vi "UHR-Fleezers Control (host) - 10.8.vi"() -> ()   [LabVIEW 2013] (continued)
  n124 = xnode "Read/Write Control"("FPGA VI Reference In"=w12, "error in"=w15, "Phase count adjustment"=w173, "Phase count adjustment (GI)"=w172, "Phase count adjustment (MCL)"=w171, "Phase Count Adjustment (APD Acq)"="Phase Adj. (APD Acq)", "Phase count adjustment (APD 1 Gate)"="Phase Adj. (APD 1 Gate)", "Phase count adjustment (APD 2 Gate)"="Phase Adj. (APD 2 Gate)", "Phase count adjustment (Green FB)"=w112, "Phase count adjustment (GI) 2"=w82) -> ("FPGA VI Reference Out"=w11:T19, "error out"=w10:errorcluster)
  n125 = call "Initialize RF boards - interlace 3.vi"("error in"=w10, "FPGA VI Reference In"=w11) -> ("FPGA VI Reference Out"=w149:T19)  [unwired: 1 out]
  n126 = call "set RF board frequency - interlace.vi"("Board 2 Frequency Limits"=w115, "Board 1 Frequency Limits"=w117, "FPGA VI Reference In"=w149, "Board 2 Frequency 3 (MHz)"="BD 2 Frequency 3 (MHz)", "Board 1 Frequency 3 (MHz)"="BD 1 Frequency 3 (MHz)", "Board 2 Frequency 2 (MHz)"="BD 2 Frequency 2 (MHz)", "Board 2 Frequency 1 (MHz)"="BD 2 Frequency 1 (MHz)", "Board 1 Frequency 2 (MHz)"="BD 1 Frequency 2 (MHz)", "Board 1 Frequency 1  (MHz)"="BD 1 Frequency 1 (MHz)") -> ("error out"=w243:errorcluster, "FPGA VI Reference Out"=w244:T19)  [unwired: 1 in]
  n127 = call "set RF board amplitude - interlace.vi"("Board 2 Amplitude Limits"=w114, "Board 1 Amplitude Limits"=w116, "error in"=w243, "FPGA VI Reference In"=w244, "Board 2 Amplitude 3 (%)"="BD 2 Amplitude 3 (%)", "Board 1 Amplitude 3 (%)"="BD 1 Amplitude 3 (%)", "Board 2 Amplitude 2 (%)"="BD 2 Amplitude 2 (%)", "Board 2 Amplitude 1 (%)"="BD 2 Amplitude 1 (%)", "Board 1 Amplitude 2 (%)"="BD 1 Amplitude 2 (%)", "Board 1 Amplitude 1 (%)"="BD 1 Amplitude 1 (%)") -> ("error out"=w8:errorcluster, "FPGA VI Reference Out"=w9:T19)
  n128 = flat-sequence {
    tunnel: w9 -> [w297]
    tunnel: w8 -> [w296]
    tunnel: [w295] -> w236
    tunnel: [w294] -> w235
    tunnel: [w301] -> w234
    tunnel: w236 -> [w301]
    tunnel: [w300] -> w233
    tunnel: w235 -> [w300]
    tunnel: w234 -> [w310]
    tunnel: w233 -> [w309]
    tunnel: [w308] -> w38
    tunnel: [w307] -> w37
    tunnel: w38 -> [w337]
    tunnel: w37 -> [w332]
    tunnel: [w337] -> w2
    tunnel: [w312] -> w1
    tunnel: [w338] -> w39
    tunnel: [w343] -> w16
    tunnel: w2 -> [w343]
    tunnel: w1 -> [w340]
    frame #0 {
      n129 = local read "Trap 1 (ON/OFF)"() -> (w289:bool)
      n130 = xnode "Read/Write Control"("FPGA VI Reference In"=w297, "error in"=w296, "Direct RF Box  Communication"=FALSE) -> ("FPGA VI Reference Out"=w295:T19, "error out"=w294:errorcluster)
      n131 = local write "Saving..."(FALSE ("Saving Data")) -> ()
      n132 = local write "Stop All"(FALSE ("Stop All")) -> ()
      n133 = local write "Index"(1.0 ("Index")) -> ()
      n134 = property on="Trap 1 ON" class="Bool (strict)"("Value"=w289) -> ()  [unwired: 2 in, 2 out]
      "Manipulating Trap" <- FALSE ("Manipulating Trap")
    }
    frame #1 {
      n135 = local read "Trap 2 (ON/OFF)"() -> (w299:bool)
      n136 = Wait (ms)(milliseconds to wait=u32 50) -> ()  [unwired: 1 out]
      n137 = property on="Trap 2 ON" class="Bool (strict)"("Val(Sgnl)"=w299) -> ()  [unwired: 2 in, 2 out]
    }
    frame #2 {
      n138 = local read "Scan Range (nm)"() -> (w303:dbl)
      n139 = xnode "Read/Write Control"("FPGA VI Reference In"=w310, "error in"=w309, "FPGA Controls  RF Box"=TRUE ("Direct RF Box  Communication")) -> ("FPGA VI Reference Out"=w308:T19, "error out"=w307:errorcluster)
      n140 = call "Update messages.vi"("Message to add"="UHR-Fleezers ready.", "Old message string"="") -> ("New message string"=w306:string)
      n141 = local write "Messages"(w306) -> ()
      n142 = property on="Scan Range (nm)" class="DigNum (strict)"("Val(Sgnl)"=w303) -> ()  [unwired: 2 in, 2 out]
    }
    frame #3 {
      w318 = T20."ASCII" ("Command")
      # "disable hysteresis\ncompensation for\nfaster performance"
      # "increase jerk\nfor faster \nresponse"
      # "disable backlash\ncompensation for\nfaster response \ntimes. necessary\nfor mouse control\nof stage"
      n143 = call "CONEX_FUNCTIONAL_GLOBAL.vi"("error in"=w332, "Command"=T20."INIT") -> ("error out"=w314:errorcluster)  [unwired: 7 in, 2 out]
      n144 = call "CONEX_FUNCTIONAL_GLOBAL.vi"("error in"=w314, "Position"=dbl[] [10.0, 12.0, 2.0], "Command"=T20."SET ULIM") -> ("error out"=w333:errorcluster)  [unwired: 6 in, 2 out]
      n145 = call "CONEX_FUNCTIONAL_GLOBAL.vi"("error in"=w333, "Position"=dbl[] [0.0, 0.0, 4.0], "Command"=T20."SET LLIM") -> ("error out"=w327:errorcluster)  [unwired: 6 in, 2 out]
      n146 = Concatenate Strings("1BA0", "\r\n") -> (w324:string)
      n147 = call "CONEX_FUNCTIONAL_GLOBAL.vi"("error in"=w327, "ASCII command"=w324, "Command"=w318) -> ("error out"=w323:errorcluster)  [unwired: 6 in, 2 out]
      n148 = Concatenate Strings("1JR0.001", "\r\n") -> (w320:string)
      n149 = call "CONEX_FUNCTIONAL_GLOBAL.vi"("error in"=w323, "ASCII command"=w320, "Command"=w318) -> ("error out"=w319:errorcluster)  [unwired: 6 in, 2 out]
      n150 = Concatenate Strings("1BH0", "\r\n") -> (w315:string)
      n151 = call "CONEX_FUNCTIONAL_GLOBAL.vi"("error in"=w319, "ASCII command"=w315, "Command"=w318) -> ("error out"=w313:errorcluster)  [unwired: 6 in, 2 out]
      n152 = call "CONEX_FUNCTIONAL_GLOBAL.vi"("error in"=w313, "Command"=T20."GET POS") -> ("error out"=w312:errorcluster, "Current Position"=w328:dbl[])  [unwired: 7 in, 1 out]
      n153 = local write "Current Position"(w328) -> ()
    }
    frame #4 {
      n154 = call "hamilton_controller.vi"("error in"=w340, "action"=T21."CONNECT") -> ("error out"=w339:errorcluster)  [unwired: 9 in]
      n155 = call "hamilton_controller.vi"("error in"=w339, "action"=T21."INITIALIZE VALVES") -> ("error out"=w338:errorcluster)  [unwired: 9 in]
    }
  }
  n156 = Subtract(x="BD 1 Frequency 1 (MHz)", y="BD 1 Frequency 2 (MHz)") -> (x-y=w159:dbl)
  n157 = Subtract(x="BD 2 Frequency 1 (MHz)", y="BD 2 Frequency 2 (MHz)") -> (x-y=w158:dbl)
  n158 = Square(x=w158) -> (x^2=w156:dbl)
  n159 = Square(x=w159) -> (x^2=w157:dbl)
  n160 = Add(x=w157, y=w156) -> (x+y=w155:dbl)
  n161 = Square Root(x=w155) -> (sqrt(x)=w154:dbl)
  n162 = local write "Trap Delta (MHz)"(w154) -> ()
  n163 = call "IMAQ Create"("Image Name"="APD 1 Image", "Image Type"=w63) -> ("New Image"=w62:T2)  [unwired: 3 in, 1 out]
  n164 = call "IMAQ Create"("Image Name"="APD 2 Image", "Image Type"=w63) -> ("New Image"=w61:T2)  [unwired: 3 in, 1 out]
  n165 = call "IMAQ Create"("Image Name"="Det. X Image", "Image Type"=w63) -> ("New Image"=w60:T2)  [unwired: 3 in, 1 out]
  n166 = call "IMAQ Create"("Image Name"="Det. Y Image", "Image Type"=w63) -> ("New Image"=w59:T2)  [unwired: 3 in, 1 out]
  n167 = Bundle("New Image"=w62, "New Image"=w61, "New Image"=w60, "New Image"=w59) -> (w58:T22)  [unwired: 1 in]
  n168 = disable-structure shown="Disabled" {
    disable-tunnel: w16 -> [w372 _]
    frame Disabled {
      w367 = T17 0 items=["Grayscale (U8)", "Grayscale (I16)", "Grayscale (SGL)", "Complex (CSG)", "RGB (U32)", "HSL (U32)", "RGB (U64)", "Grayscale (U16)"] ("Image Type")
      n169 = call <vilib>:"IMAQ Init.vi"("Interface Name"="img0") -> ("error out"=w369:errorcluster, "IMAQ Session Out"=w371:refnum<k11>)  [unwired: 9 in]
      n170 = call <vilib>:"IMAQ Grab Setup.vi"("error in (no error)"=w369, "IMAQ Session In"=w371) -> ("error out"=w365:errorcluster, "IMAQ Session Out"=w366:refnum<k11>)  [unwired: 8 in]
      n171 = call "IMAQ Create"("Image Name"="untitled", "Image Type"=w367) -> ("New Image"=w364:T2)  [unwired: 3 in, 1 out]
      n172 = call <vilib>:"Application Directory.vi"() -> ("Application Directory"=w351:path)
      n173 = Build Path(base path=w351, name or relative path="_trap_screen_positions") -> (appended path=w359:path)
      n174 = Open/Create/Replace File(file path (use dialog)=w359, operation (0:open)=T23."open or create", access (0:read/write)=enum16{"read/write", "read-only", "write-only"}."read/write") -> (refnum out=w361:refnum<file>)  [unwired: 3 in, 2 out]
      n175 = local read "Trap Sets"() -> (w353:u32)
      n176 = for "Load trap positions on video screen from file." {
        N: w353 -> [_]
        tunnel: [w379] -> w354
        tunnel: w361 -> [w378]
        tunnel: [w375] -> w350 mode=indexing
        w377 = 4
        n177 = for {
          N: w377 -> [_]
          tunnel: [w383] -> w379
          tunnel: w378 -> [w382]
          tunnel: w377 -> [w381]
          tunnel: [w380] -> w376 mode=indexing
          n178 = Read from Binary File(5:w381, 11:w382) -> (2:w380:i32, 3:w383:refnum<file>)  [unwired: 4 in, 2 out]
        }
        n179 = Array To Cluster(array=w376) -> (cluster=w375:T27)
      }
      n180 = node-c288() -> (w374:T24)  [unwired: 4 in]
      n181 = timed-loop "acquire video and stage position" {
        timing: w374 -> [_]
        timing-out: [_] -> w373
        tunnel: w366 -> [w402]
        tunnel: w365 -> [w401]
        tunnel: w364 -> [w400]
        tunnel: [w399] -> w346
        tunnel: [w396] -> w347
        tunnel: [w397] -> w345
        tunnel: w372 -> [_]
        shift-right: [w393] -> w363
        shift-left: w350 -> [w394]
        tunnel: w353 -> [w391]
        stop <- w398 stop-if-true
        n182 = node-c288() -> ()  [unwired: 1 in, 1 out]
        n183 = event shown="[2] \"Primary Video Display\": Mouse Down" {
          selector: _ -> [_ _ _ _]
          dyn-events: _ -> [_ _ _ _]
          timeout: 10 -> [_ _ _ _]
          tunnel: w402 -> [w413 w428 w437 w456]
          tunnel: w401 -> [w412 w430 w435 w458]
          tunnel: w400 -> [w411 w429 w436 w457]
          tunnel: [w410 w428 w437 w456] -> w399
          tunnel: [w403 w432 FALSE FALSE] -> w398
          tunnel: [w407 w430 w435 w458] -> w397
          tunnel: [w406 w429 w436 w457] -> w396
          tunnel: "radius" -> [_ _ w442 _]
          tunnel: w394 -> [w404 w431 w440 _]
          tunnel: [w404 w431 w441 cluster{i32, i32, i32, i32}[] []] -> w393
          tunnel: w391 -> [_ _ w433 _]
          event Timeout {
            n184 = event-data() -> ()  [unwired: 1 in, 2 out]
            n185 = call <vilib>:"IMAQ Grab Acquire.vi"("error in (no error)"=w412, "Image In"=w411, "IMAQ Session In"=w413) -> ("error out"=w408:errorcluster, "Image Out"=w409:T2, "IMAQ Session Out"=w410:refnum<k11>)  [unwired: 5 in, 1 out]
            n186 = case shown="True" "trap\nmarkers?" {
              tunnel: w404 -> [_ w421]
              tunnel: w409 -> [w415 w420]
              tunnel: w408 -> [w414 w419]
              tunnel: [w414 w418] -> w407
              tunnel: [w415 w416] -> w406
              frame False {
              }
              frame True {
                n187 = for {
                  tunnel: w421 -> [w427] mode=indexing
                  shift-right: [w425] -> w416
                  shift-left: w420 -> [w426]
                  tunnel: w419 -> [w424]
                  tunnel: [w423] -> w418
                  tunnel: u32 16711680 ("Color") -> [w422]
                  n188 = call "IMAQ Overlay Oval"("Color"=w422, "error in (no error)"=w424, "Bounding Rectangle"=w427, "Image"=w426) -> ("error out"=w423:errorcluster, "Image Out"=w425:T2)  [unwired: 6 in]
                }
              }
            }
            "Primary Video Display" <- w406
            n189 = Unbundle By Name(w408) -> ("status"=w403:bool)
          }
          event "Stop All": Value Change {
            n190 = event-data() -> ()  [unwired: 1 in, 5 out]
            n191 = local read "Stop All"() -> (w432:bool)
          }
          event "Primary Video Display": Mouse Down {
            n192 = event-data() -> ()  [unwired: 1 in, 7 out]
            n193 = Array Size(array=w440) -> (size(s)=w439:i32)
            n194 = Less?(x=w439, y=w433) -> (x < y?=w438:bool)
            n195 = case shown="True" w438 {
              tunnel: w442 -> [_ w452]
              tunnel: w440 -> [w443 w446]
              tunnel: [w443 w445] -> w441
              frame False {
              }
              frame True {
                n196 = property on="Primary Video Display" class="ImageControl"() -> ("Last Mouse Position"=w444:cluster{"X":i32, "Y":i32})  [unwired: 2 in, 2 out]
                n197 = Unbundle By Name(w444) -> ("X"=w454:i32, "Y"=w453:i32)
                n198 = Add(x=w453, y=w452) -> (x+y=w450:i32)
                n199 = Subtract(x=w453, y=w452) -> (x-y=w448:i32)
                n200 = Add(x=w454, y=w452) -> (x+y=w449:i32)
                n201 = Subtract(x=w454, y=w452) -> (x-y=w451:i32)
                n202 = Bundle(w451, w450, w449, w448) -> (w447:cluster{i32, i32, i32, i32})  [unwired: 1 in]
                n203 = Build Array (concatenate)(w446, w447) -> (w445:T28)
              }
            }
          }
          event "clear markers": Value Change {
            n204 = event-data() -> ()  [unwired: 1 in, 5 out]
          }
        }
        n205 = node-c288() -> ()  [unwired: 1 in, 1 out]
      }
      n206 = node-c288(w373) -> ()  [unwired: 1 out]
      n207 = Set File Position(offset (in bytes) (0)=i64 0, refnum=w354, from (0:start)=enum16{"start", "end", "current"}."start") -> (refnum out=w355:refnum<file>)  [unwired: 1 in, 1 out]
      n208 = for "Write trap positions to file so they can be remembered\nwhen program is removed from memory" {
        tunnel: w363 -> [w387] mode=indexing
        tunnel: [w385] -> w362
        tunnel: w355 -> [w384]
        n209 = Cluster To Array(cluster=w387) -> (array=w386:i32[])
        n210 = for {
          tunnel: w386 -> [w390] mode=indexing
          tunnel: [w389] -> w385
          tunnel: w384 -> [w388]
          n211 = Write to Binary File(file (use dialog)=w388, data=w390) -> (refnum out=w389:refnum<file>)  [unwired: 4 in, 2 out]
        }
      }
      n212 = Close File(refnum=w362) -> ()  [unwired: 1 in, 2 out]
      n213 = call "IMAQ Dispose"("Image"=w347, "error in (no error)"=w345) -> ("error out"=w344:errorcluster)  [unwired: 4 in]
      n214 = call <vilib>:"IMAQ Stop.vi"("error in (no error)"=w344, "IMAQ Session In"=w346) -> ("error out"=w348:errorcluster, "IMAQ Session Out"=w349:refnum<k11>)  [unwired: 8 in]
      n215 = call <vilib>:"IMAQ Close.vi"("error in (no error)"=w348, "IMAQ Session In"=w349) -> ()  [unwired: 9 in, 1 out]
    }
    frame Enabled {
    }
  }
  n216 = call <vilib>:"Initialize Mouse.vi"() -> ("error out"=w18:errorcluster, "device ID"=w19:refnum<k1>)  [unwired: 10 in]
  n217 = node-c288() -> (w4:T24)  [unwired: 4 in]
  n218 = call-poly <vilib>:"Acquire Input Data.vi"("device ID"=w19, "error in (no error)"=w18) -> ("device ID"=w20:refnum<k1>, "error out"=w17:errorcluster)  [unwired: 14 in, 2 out]
  n219 = timed-loop {
    tunnel: w20 -> [w471]
    tunnel: [w470] -> w21
    tunnel: [w469] -> _
    tunnel: w17 -> [w468]
    tunnel: w16 -> [_]
    shift-right: ["Use mouse to move stage\n(press mouse wheel to quit)"] -> _
    shift-left: _ -> [w465]
    timing: w4 -> [_]
    timing-out: [_] -> w3
    i -> [w464]
    stop <- w467 stop-if-true
    n220 = node-c288() -> ()  [unwired: 1 in, 1 out]
    n221 = case shown="False" "Use mouse to move stage\n(press mouse wheel to quit)" {
      tunnel: w471 -> [w481 w499]
      tunnel: [w481 w522] -> w470
      tunnel: [w474 w503] -> w469
      tunnel: w468 -> [w475 w497]
      tunnel: w465 -> [_ w500]
      tunnel: w464 -> [_ w495]
      frame False {
        n222 = case shown="True" "reset motor comm. link" {
          tunnel: [w482 w485] -> w476
          tunnel: w475 -> [w482 w484]
          frame False {
          }
          frame True {
            n223 = call "CONEX_FUNCTIONAL_GLOBAL.vi"("error in"=w484, "Command"=T20."CLOSE") -> ("error out"=w487:errorcluster)  [unwired: 7 in, 2 out]
            n224 = flat-sequence {
              tunnel: w487 -> [w490]
              tunnel: [w490] -> w486
              frame #0 {
                n225 = Wait (ms)(milliseconds to wait=u32 50) -> ()  [unwired: 1 out]
              }
            }
            n226 = local write "reset motor comm. link"(FALSE ("reset motor comm. link")) -> ()
            n227 = call "CONEX_FUNCTIONAL_GLOBAL.vi"("error in"=w486, "Command"=T20."INIT") -> ("error out"=w485:errorcluster)  [unwired: 7 in, 2 out]
          }
        }
        n228 = call "CONEX_FUNCTIONAL_GLOBAL.vi"("Axis"=enum16{"X", "Y", "Z", "XY", "XZ", "YZ", "XYZ"}."XYZ", "error in"=w476, "Command"=T20."GET POS") -> ("error out"=w474:errorcluster, "Current Position"=w478:dbl[])  [unwired: 6 in, 1 out]
        n229 = local write "Current Position"(w478) -> ()
      }
      frame True {
        # "put cursor somewhere\nwhere mouse clicks and \nmouse wheel moves won't\nbe heard by the window"
        n230 = Not(x=w500) -> (.not. x?=w501:bool)
        n231 = Quotient & Remainder(x=w495, y=10) -> (x-y*floor(x/y)=w493:i32)  [unwired: 1 out]
        n232 = case shown="True" w501 {
          tunnel: w499 -> [w526 w530]
          tunnel: [w526 w529] -> w498
          tunnel: w497 -> [w525 w528]
          tunnel: [w525 w527] -> w496
          frame False {
          }
          frame True {
            n233 = call-poly <vilib>:"Acquire Input Data.vi"("device ID"=w530, "error in (no error)"=w528) -> ("device ID"=w529:refnum<k1>, "error out"=w527:errorcluster)  [unwired: 14 in, 2 out]
          }
        }
        n234 = Equal To 0?(x=w493) -> (x = 0?=w492:bool)
        n235 = case shown="True" w492 {
          frame False {
          }
          frame True {
            # "SetCursorPos"
            n236 = dll-call lib="User32.dll" fn="SetCursorPos"(900, 600) -> ()  [unwired: 5 in, 3 out]
          }
        }
        n237 = call-poly <vilib>:"Acquire Input Data.vi"("device ID"=w498, "key mode"=enum16{"RELATIVE", "ABSOLUTE"}."RELATIVE", "error in (no error)"=w496) -> ("device ID"=w522:refnum<k1>, "axis info"=w520:T29, "error out"=w502:errorcluster)  [unwired: 13 in, 1 out]
        n238 = Cluster To Array(cluster=w520) -> (array=w518:i32[])
        n239 = Compound Arithmetic op=MULTIPLY(invert 10000.0 ("value"), "mouse sensitivity", w518) -> (w516:dbl[])
        n240 = call "subVI_explode3array.vi"("Array"=w516) -> ("x"=w507:dbl, "y"=w506:dbl, "z"=w515:dbl)  [unwired: 12 in]
        n241 = case shown="False" "invert y?" {
          tunnel: w506 -> [w531 w533]
          tunnel: [w531 w532] -> w505
          frame False {
          }
          frame True {
            n242 = Negate(x=w533) -> (-x=w532:dbl)
          }
        }
        n243 = case shown="False" "invert x?" {
          tunnel: w507 -> [w534 w536]
          tunnel: [w534 w535] -> w504
          frame False {
          }
          frame True {
            n244 = Negate(x=w536) -> (-x=w535:dbl)
          }
        }
        n245 = Divide(x=w515, y=50.0) -> (x/y=w513:dbl)
        n246 = Build Array(w504, w505, w513) -> (w510:dbl[])
        n247 = call "CONEX_FUNCTIONAL_GLOBAL.vi"("Axis"=enum16{"X", "Y", "Z", "XY", "XZ", "YZ", "XYZ"}."XYZ", "error in"=w502, "Position"=w510, "Command"=T20."REL MOVE") -> ("error out"=w503:errorcluster)  [unwired: 5 in, 2 out]
      }
    }
    n248 = local read "Stop All"() -> (w467:bool)
    n249 = node-c288() -> ()  [unwired: 1 in, 1 out]
  }
  n250 = node-c288(2 ("Processor")) -> (w7:T24)  [unwired: 3 in]
  n251 = node-c288() -> (w68:T24)  [unwired: 4 in]
  n252 = node-c288(i64 1 ("Period"), 1 ("Processor")) -> (w163:T24)  [unwired: 2 out]
  n253 = disable-structure shown="Enabled" {
    disable-tunnel: [w538 _] -> w32
    disable-tunnel: w16 -> [w537 _]
    frame Enabled {
      n254 = node-c288() -> (w540:T24)  [unwired: 4 out]
      n255 = timed-loop "Rough control of MCL mirror stage (debugging)" {
        tunnel: w537 -> [w543]
        tunnel: [w542] -> w538
        timing: w540 -> [_]
        timing-out: [_] -> w539
        stop <- w542 stop-if-true
        n256 = node-c288() -> ()  [unwired: 2 out]
        n257 = case shown="1" "MCL Mode" {
          tunnel: w543 -> [_ w546 w593]
          frame 0, Default {
            # "manual positioning"
          }
          frame 1 {
            # "sinusoidal wave"
            n258 = node-c288() -> (w548:T24)  [unwired: 4 out]
            n259 = timed-loop "Oscillate MCL mirror" {
              timing: w548 -> [_]
              timing-out: [_] -> w547
              tunnel: w546 -> [w587]
              i -> [w586]
              stop <- w549 stop-if-true
              n260 = node-c288() -> (w585:i64)  [unwired: 1 out]
              n261 = Multiply(x="AO1", y=32767.0) -> (x*y=w581:dbl)
              n262 = Multiply(x="AO2", y=32767.0) -> (x*y=w576:dbl)
              n263 = Divide(x=w581, y=10.0) -> (x/y=w582:dbl)
              n264 = Divide(x=w576, y=10.0) -> (x/y=w577:dbl)
              n265 = To Word Integer(number=w582) -> (16bit integer=w574:i16)
              n266 = To Word Integer(number=w577) -> (16bit integer=w573:i16)
              n267 = Divide(x=w585, y=i64 1000) -> (x/y=w556:dbl)
              n268 = Multiply(x=w556, y=w586) -> (x*y=w567:dbl)
              n269 = Multiply(x="Osc. freq. (Hz) 2", y=6.283185307179586) -> (x*y=w568:dbl)
              n270 = Multiply(x=w568, y=w567) -> (x*y=w566:dbl)
              n271 = Sine(x=w566) -> (sin(x)=w565:dbl)
              n272 = Multiply(x=w565, y="Osc. amp. (V)") -> (x*y=w563:dbl)
              n273 = Add(x=w563, y="Osc. center (V)") -> (x+y=w561:dbl)
              n274 = Divide(x=w561, y=10.0) -> (x/y=w559:dbl)
              n275 = Multiply(x=w559, y=32767.0) -> (x*y=w554:dbl)
              n276 = Select(t=w554, s="Scan axis", f=w574) -> (s? t:f=w572:dbl)
              n277 = Select(t=w573, s="Scan axis", f=w554) -> (s? t:f=w571:dbl)
              n278 = local read "MCL Mode"() -> (w553:u16)
              n279 = Not Equal?(x=w553, y=u16 1) -> (x != y?=w550:bool)
              n280 = local read "Stop All"() -> (w551:bool)
              n281 = xnode "Read/Write Control"("FPGA VI Reference In"=w587, "AO1"=w572, "AO2"=w571) -> ()  [unwired: 1 in, 2 out]
              n282 = Compound Arithmetic op=OR(w551, w550) -> (w549:bool)
              n283 = node-c288() -> ()  [unwired: 2 out]
            }
            n284 = node-c288(w547) -> ()  [unwired: 1 out]
          }
          frame 2 {
            # "linear scan"
            n285 = case shown="True" "Start Scan" {
              tunnel: w593 -> [_ w605]
              frame False {
              }
              frame True {
                n286 = Subtract(x="End (V)", y="Begin (V)") -> (x-y=w601:dbl)
                n287 = Decrement(x="N Points") -> (x-1=w600:dbl)
                n288 = Divide(x=w601, y=w600) -> (x/y=w598:dbl)
                n289 = for {
                  N: "N Points" -> [_]
                  tunnel: "Begin (V)" -> [w618]
                  tunnel: w605 -> [w610]
                  tunnel: [w609] -> w604 mode=indexing
                  tunnel: w598 -> [w608]
                  tunnel: [w606] -> w597 mode=indexing
                  i -> [w617]
                  n290 = Multiply(x=w608, y=w617) -> (x*y=w616:dbl)
                  n291 = Add(x=w618, y=w616) -> (x+y=w613:dbl)
                  n292 = local read "Scan axis"() -> (w607:bool)
                  n293 = local read "AO1"() -> (w615:dbl)
                  n294 = local read "AO2"() -> (w614:dbl)
                  n295 = Select(t=w613, s=w607, f=w615) -> (s? t:f=w612:dbl)
                  n296 = Select(t=w614, s=w607, f=w613) -> (s? t:f=w611:dbl)
                  n297 = flat-sequence {
                    tunnel: w612 -> [w622]
                    tunnel: w611 -> [w621]
                    tunnel: w610 -> [w619]
                    tunnel: [w632] -> w609
                    tunnel: [w631] -> w606
                    frame #0 {
                      w625 = 10.0 ("y")
                      w620 = 32767.0 ("y")
                      n298 = Multiply(x=w622, y=w620) -> (x*y=w628:dbl)
                      n299 = Multiply(x=w621, y=w620) -> (x*y=w626:dbl)
                      n300 = Divide(x=w628, y=w625) -> (x/y=w629:dbl)
                      n301 = Divide(x=w626, y=w625) -> (x/y=w627:dbl)
                      n302 = To Word Integer(number=w629) -> (16bit integer=w623:i16)
                      n303 = To Word Integer(number=w627) -> (16bit integer=w624:i16)
                      n304 = xnode "Read/Write Control"("FPGA VI Reference In"=w619, "AO1"=w623, "AO2"=w624) -> ()  [unwired: 1 in, 2 out]
                    }
                    frame #1 {
                      n305 = Wait (ms)(milliseconds to wait="DAQ Delay (ms)") -> ()  [unwired: 1 out]
                    }
                    frame #2 {
                      n306 = local read "Slow mean"() -> (w632:dbl)
                      n307 = local read "Sigma"() -> (w631:dbl)
                    }
                  }
                }
                n308 = Bundle("Begin (V)"="Begin (V)", w598, w604) -> (→"MCL Scan":cluster{"Begin (V)":dbl, dbl, dbl[]})  [unwired: 1 out]
                n309 = Bundle("Begin (V)"="Begin (V)", w598, w597) -> (→"MCL Scan 2":cluster{"Begin (V)":dbl, dbl, dbl[]})  [unwired: 1 out]
              }
            }
          }
        }
        n310 = local read "Stop All"() -> (w542:bool)
        n311 = node-c288() -> ()  [unwired: 2 out]
      }
      n312 = node-c288(w539) -> ()  [unwired: 1 out]
    }
    frame Disabled {
    }
  }
  n313 = timed-loop "Control parameters (event loop)" {
    tunnel: w16 -> [w638]
    shift-right: [w637] -> _
    shift-left: errorcluster {"status"=FALSE, "code"=0, "source"=""} ("error out") -> [w636]
    tunnel: [w635] -> w34
    timing: w7 -> [_]
    timing-out: [_] -> w6
    stop <- w635 stop-if-true
    n314 = node-c288() -> ()  [unwired: 1 in, 1 out]
    n315 = event shown="[32] \"Raster Scanning...\": Value Change" {
      selector: _ -> [_ _ _ _ _ _ _ _ _ _ _ _ _ _ _ _ _ _ _ _ _ _ _ _ _ _ _ _ _ _ _ _ _ _ _ _ _ _ _ _ _ _ _ _ _ _ _ _ _ _ _ _ _ _ _ _ _]
      dyn-events: _ -> [_ _ _ _ _ _ _ _ _ _ _ _ _ _ _ _ _ _ _ _ _ _ _ _ _ _ _ _ _ _ _ _ _ _ _ _ _ _ _ _ _ _ _ _ _ _ _ _ _ _ _ _ _ _ _ _ _]
      timeout: _ -> [_ _ _ _ _ _ _ _ _ _ _ _ _ _ _ _ _ _ _ _ _ _ _ _ _ _ _ _ _ _ _ _ _ _ _ _ _ _ _ _ _ _ _ _ _ _ _ _ _ _ _ _ _ _ _ _ _]
      tunnel: w638 -> [w676 _ _ _ w713 _ w735 _ w799 _ _ _ w842 _ _ w885 w891 w896 w902 w938 w956 w963 _ w981 w992 w1003 w1014 w1025 w1036 w1054 w1060 w1154 _ w1163 w1201 _ _ w1300 w1304 w1315 w1319 w1323 _ w1331 _ _ _ _ w1465 _ w1482 w1485 w1494 w1497 w1501 _ w1518]
      tunnel: [w675 _ _ _ w703 _ w734 _ w762 _ w807 _ w821 _ _ w884 w887 w893 w899 w937 w954 w962 _ w975 w986 w997 w1008 w1019 w1030 w1052 w1059 w1152 _ w1161 w1199 _ _ w1298 w1302 w1305 w1317 w1321 _ w1329 _ _ _ _ w1463 _ _ _ _ _ _ _ _] -> w637
      tunnel: w636 -> [w674 _ _ _ w712 _ w733 _ w794 _ w807 _ w841 _ _ w883 w886 w892 w898 w936 w955 w961 _ w980 w991 w1002 w1013 w1024 w1035 w1053 w1058 w1153 _ w1162 w1200 _ _ w1299 w1303 w1314 w1318 w1322 _ w1330 _ _ _ _ w1464 _ w1481 w1484 w1493 w1496 w1500 _ w1517]
      tunnel: [_ _ _ _ _ _ _ _ _ _ w806 _ _ _ _ _ _ _ _ _ _ _ _ _ _ _ _ _ _ _ _ _ _ _ _ _ _ _ _ _ _ _ _ _ _ _ _ _ _ _ _ _ _ _ _ _ _] -> w635
      tunnel: [_ _ _ _ _ _ _ "Round T1 X" _ _ _ _ _ _ _ _ _ _ _ _ _ _ _ _ _ _ _ _ _ _ _ _ _ _ _ _ _ _ _ _ _ _ _ _ _ _ _ _ _ _ _ _ _ _ _ _ _] -> _
      tunnel: [_ _ _ "Adjust Scale\nto Mean" _ _ _ _ _ _ _ _ _ _ _ _ _ _ _ _ _ _ _ _ _ _ _ _ _ _ _ _ _ _ _ _ _ _ _ _ _ _ _ _ _ _ _ _ _ _ _ _ _ _ "Set SP to Reading" _ _] -> _
      tunnel: [_ _ _ _ _ _ _ _ _ "Round T2 X" _ "Delayed Interlace Start" _ _ _ _ _ _ _ _ _ _ _ _ _ _ _ _ _ _ _ _ _ _ _ _ _ _ _ _ _ _ _ _ _ _ _ _ _ _ _ _ _ _ _ _ _] -> _
      event "AI Count (ticks)", "Sets to FIFO (Traps)", "Save ave N", "FPGA Ave.", "# Samples/channel", "N sets to save": Value Change {
        # "So that if 'Save ave N' is updated, the AOD scanning code updates too."
        n316 = event-data() -> ()  [unwired: 6 out]
        n317 = local read "AI Count (ticks)"() -> (w656:u32)
        n318 = Boolean To (0,1)(Boolean="Sets to FIFO (Traps)") -> (0, 1=w666:cluster{"Set 1":i16, "Set 2":i16, "Set 3":i16})
        n319 = xnode "Read/Write Control"("FPGA VI Reference In"=w676, "error in"=w674, "ai count"=w656, "AI1 Sets to FIFO"="Sets to FIFO (Traps)", "N of AI1 Int Acq Sets"="N Acq Sets (Traps + Fl.)") -> ("error out"=w675:errorcluster)  [unwired: 1 out]
        n320 = Cluster To Array(cluster=w666) -> (array=w665:i16[])
        n321 = To Unsigned Long Integer(number=w665) -> (unsigned 32bit integer=w645:u32[])
        n322 = local read "Scan steps (AOD)"() -> (w667:u64)
        n323 = Multiply(x=w656, y="N Acq Sets (Traps + Fl.)") -> (x*y=w654:u32)
        n324 = Divide(x=40000000.0, y=w656) -> (x/y=w648:dbl)
        "AI rate (Hz)" <- w648
        "Ave. Rate (Hz)" <- w648
        n325 = Add Array Elements(numeric array=w645) -> (sum=w657:u32)
        "Trap Sets" <- w657
        n326 = Reciprocal(x=w648) -> (1/x=→"Ave. Period (s)":dbl)
        n327 = property on="Scan steps (AOD)" class="DigNum (strict)"("Val(Sgnl)"=w667) -> ()  [unwired: 2 in, 2 out]
        n328 = Divide(x=w648, y="N Acq Sets (Traps + Fl.)") -> (x/y=w671:dbl)
        "Data Rate (Hz)" <- w671
        n329 = Reciprocal(x=w671) -> (1/x=→"Data Period (s)":dbl)
        n330 = local read "Save ave N"() -> (w670:dbl)
        n331 = Divide(x=w671, y=w670) -> (x/y=w669:dbl)
        "Save Data Rate (Hz)" <- w669
        n332 = Reciprocal(x=w669) -> (1/x=→"Save Data Period (s)":dbl)
        n333 = Multiply(x=w654, y="# Samples/trap") -> (x*y=w652:u32)
        "Counts/DMA" <- w652
        n334 = property on="Trap Disp. Downsample" class="DigNum (strict)"("Maximum"="# Samples/trap") -> ()  [unwired: 2 in, 2 out]
        n335 = Multiply(x=w657, y="# Samples/trap") -> (x*y=w646:u32)
        "# Samples/channel" <- w646
        n336 = Multiply(x=w646, y=u32 8) -> (x*y=→"Trap AI Elements/DMA read":u32)
        n337 = local read "APD Int. Count"() -> (w653:u32)
        n338 = Multiply(x=w646, y=u32 3) -> (x*y=→"Trap Pos Elements/DMA read":u32)
        n339 = Divide(x=w652, y=w653) -> (x/y=w643:dbl)
        "APD Samples/FIFO Acq." <- w643
        n340 = Divide(x=w652, y=40000000.0) -> (x/y=w650:dbl)
        "DMA Update Period (s)" <- w650
        n341 = Multiply(x=2.0, y=w643) -> (x*y=→"APD Elements/DMA read":dbl)
        n342 = property on="APD Disp. Downsample" class="DigNum (strict)"("Maximum"=w643) -> ()  [unwired: 2 in, 2 out]
        n343 = local read "N sets to save"() -> (w663:u32)
        n344 = Multiply(x=w650, y=w663) -> (x*y=→"Total Time (s)":dbl)
        "FPGA Averaging" <- FALSE ("FPGA Averaging")
      }
      event "Rescale on Mean": Value Change {
        n345 = event-data() -> ()  [unwired: 7 out]
        n346 = And(x=FALSE, y="Rescale on Mean") -> (x .and. y?=w678:bool)
        n347 = local write "Rescale on Mean"(w678) -> ()
        n348 = local read "Bead Mean (nm)"() -> (w683:dbl)
        n349 = Add(x="Amplitude (nm)", y=w683) -> (x+y=w681:dbl)
        n350 = Subtract(x=w683, y="Amplitude (nm)") -> (x-y=w680:dbl)
        n351 = property on="Bead Separation" class="WFChart (strict)"("YScale.Minimum"=w680) -> ()  [unwired: 2 in, 2 out]
        n352 = property on="Bead Separation" class="WFChart (strict)"("YScale.Maximum"=w681) -> ()  [unwired: 2 in, 2 out]
      }
      event "Detector Type": Value Change {
        n353 = event-data() -> ()  [unwired: 7 out]
        n354 = local read "AI labels"() -> (w684:string[])
        n355 = property on="High Res. Display" class="Ring (strict)"("Strings []"=w684) -> ()  [unwired: 2 in, 2 out]
        n356 = Build Array (concatenate)(w684, "none") -> (w685:string[])
        n357 = property on="FFT 1 Choice 1" class="Ring (strict)"("Strings []"=w685) -> ()  [unwired: 2 in, 2 out]
        n358 = property on="FFT 1 Choice 2" class="Ring (strict)"("Strings []"=w685) -> ()  [unwired: 2 in, 2 out]
        n359 = property on="FFT 2 Choice 1" class="Ring (strict)"("Strings []"=w685) -> ()  [unwired: 2 in, 2 out]
        n360 = property on="FFT 2 Choice 2" class="Ring (strict)"("Strings []"=w685) -> ()  [unwired: 2 in, 2 out]
        n361 = Bundle("APD 1", "APD 2") -> (w688:cluster{string, string})  [unwired: 1 out]
        n362 = Cluster To Array(cluster=w688) -> (array=w686:string[])
        n363 = Build Array (concatenate)(w686, w685) -> (w690:string[])
        n364 = Array Size(array=w690) -> (size(s)=w691:i32)
        n365 = property on="Signals to Plot" class="LstBox (strict)"("Item Names"=w690) -> ()  [unwired: 2 in, 2 out]
        n366 = property on="Signals to Plot" class="LstBox (strict)"("Number of Rows"=w691) -> ()  [unwired: 2 in, 2 out]
        n367 = property on="All Signals" class="WFChart (strict)"("LegNumRows"=w691) -> ()  [unwired: 2 in, 2 out]
      }
      event "Adjust Scale\nto Mean": Value Change {
        n368 = event-data() -> ()  [unwired: 7 out]
        n369 = local read "APD 1 Rate (Hz)"() -> (w700:dbl)
        n370 = Multiply(x=1000.0, y="Above (kHz)") -> (x*y=w698:dbl)
        n371 = Multiply(x=1000.0, y="Below (kHz)") -> (x*y=w696:dbl)
        n372 = Add(x=w698, y=w700) -> (x+y=w693:dbl)
        n373 = Subtract(x=w700, y=w696) -> (x-y=w694:dbl)
        n374 = property on="APD Chart" class="WFChart (strict)"("YScale.Minimum"=w694) -> ()  [unwired: 2 in, 2 out]
        n375 = property on="APD Chart" class="WFChart (strict)"("YScale.Maximum"=w693) -> ()  [unwired: 2 in, 2 out]
      }
      event "Phase adj. (AI1)", "+ phase (AI1)", "- phase (AI1)": Value Change {
        n376 = event-data() -> ()  [unwired: 7 out]
        n377 = Negate(x="Phase adj. (AI1)") -> (-x=w710:i16)
        n378 = Select(t=w710, s="- phase (AI1)", f="Phase adj. (AI1)") -> (s? t:f=w709:i16)
        n379 = xnode "Read/Write Control"("FPGA VI Reference In"=w713, "error in"=w712, "Phase count adjustment"=w709) -> ("FPGA VI Reference Out"=w708:T19, "error out"=w707:errorcluster)
        n380 = Or(x="- phase (AI1)", y="+ phase (AI1)") -> (x .or. y?=w704:bool)
        n381 = xnode "Read/Write Control"("FPGA VI Reference In"=w708, "error in"=w707, "+ phase"=w704) -> ("error out"=w703:errorcluster)  [unwired: 1 out]
      }
      event "Signals to Plot": Double Click {
        w716 = u32 9868950 ("Color Box")
        n382 = event-data() -> ("Row"=w718:i32)  [unwired: 9 out]
        n383 = property on="All Signals" class="WFChart (strict)"("Active Plot"=w718) -> (error out=w729:errorcluster)  [unwired: 2 in, 1 out]
        n384 = property on="All Signals" class="WFChart (strict)" props=["Plot", "Visible?", "Plot", "Plot Color"](error in=w729) -> (error out=w728:errorcluster, "Plot.Visible?"=w727:bool)  [unwired: 1 in, 2 out]
        n385 = Select(t=FALSE ("Plot.Visible"), s=w727, f=TRUE ("Plot.Visible")) -> (s? t:f=w722:bool)
        n386 = property on="All Signals" class="WFChart (strict)"(error in=w728, "Plot.Visible?"=w722) -> (error out=w724:errorcluster)  [unwired: 1 in, 1 out]
        n387 = property on="All Signals" class="WFChart (strict)"(error in=w724) -> (error out=w719:errorcluster, "Plot.Plot Color"=w723:u32)  [unwired: 1 in, 1 out]
        n388 = property on="Signals to Plot" class="LstBox (strict)"(error in=w719, "Active Row"=w718) -> (error out=w717:errorcluster)  [unwired: 1 in, 1 out]
        n389 = Select(t=w723, s=w722, f=u32 0) -> (s? t:f=w720:u32)
        n390 = property on="Signals to Plot" class="LstBox (strict)"(error in=w717, "CellFontColor"=w720, "SelColor"=w716, "CellBG"=w716, "CellFontSize"=u32 20 ("Active Row:Cell Font:Size"), "CellFontBold"=TRUE ("Active Row:Cell Font:Bold")) -> ()  [unwired: 1 in, 2 out]
      }
      event "BD 1 Frequency 1 (MHz)", "BD 1 Frequency 2 (MHz)", "BD 1 Frequency 3 (MHz)", "BD 2 Frequency 1 (MHz)", "BD 2 Frequency 2 (MHz)", "BD 2 Frequency 3 (MHz)", "Trap Delta (MHz)": Value Change {
        # "anytime one of the frequencies is changed, write it to the RF board UNLESS Set 2 is being oscillated. The oscillation\nscript writes the frequencies to the RF board."
        n391 = event-data() -> ("CtlRef"=w732:refnum<vi>)  [unwired: 6 out]
        n392 = control-ref of="Trap Delta (MHz)"() -> (w731:refnum<vi>)
        n393 = Equal?(x=w731, y=w732) -> (x = y?=w730:bool)
        n394 = case shown="False" "Oscillate Set 2" {
          tunnel: w735 -> [w755 _]
          tunnel: [w754 w758] -> w734
          tunnel: w733 -> [w753 w758]
          tunnel: w730 -> [w739 _]
          frame False {
            n395 = local read "BD 1 Frequency 1 (MHz)"() -> (w737:dbl)
            n396 = local read "BD 1 Frequency 2 (MHz)"() -> (w741:dbl)
            n397 = Add(x=w737, y="Trap Delta (MHz)") -> (x+y=w740:dbl)
            n398 = Select(t=w740, s=w739, f=w741) -> (s? t:f=w738:dbl)
            n399 = local read "Y RF Frequency Limits (MHz)"() -> (w743:T16)
            n400 = local read "X RF Frequency Limits (MHz)"() -> (w744:T16)
            n401 = local read "BD 1 Frequency 3 (MHz)"() -> (w756:dbl)
            n402 = local write "BD 1 Frequency 2 (MHz)"(w738) -> ()
            n403 = local read "BD 2 Frequency 1 (MHz)"() -> (w747:dbl)
            n404 = local read "BD 2 Frequency 2 (MHz)"() -> (w746:dbl)
            n405 = local read "BD 2 Frequency 3 (MHz)"() -> (w757:dbl)
            n406 = call "set RF board frequency - interlace.vi"("Board 2 Frequency Limits"=w743, "Board 1 Frequency Limits"=w744, "error in"=w753, "FPGA VI Reference In"=w755, "Board 2 Frequency 3 (MHz)"=w757, "Board 1 Frequency 3 (MHz)"=w756, "Board 2 Frequency 2 (MHz)"=w746, "Board 2 Frequency 1 (MHz)"=w747, "Board 1 Frequency 2 (MHz)"=w738, "Board 1 Frequency 1  (MHz)"=w737) -> ("error out"=w754:errorcluster)  [unwired: 1 out]
            n407 = Subtract(x=w747, y=w746) -> (x-y=w751:dbl)
            n408 = Subtract(x=w738, y=w737) -> (x-y=w752:dbl)
            n409 = Square(x=w751) -> (x^2=w749:dbl)
            n410 = Square(x=w752) -> (x^2=w750:dbl)
            n411 = Add(x=w750, y=w749) -> (x+y=w748:dbl)
            n412 = Square Root(x=w748) -> (sqrt(x)=w745:dbl)
            n413 = local write "Trap Delta (MHz)"(w745) -> ()
            n414 = property on="Initial delta (MHz)" class="DigNum (strict)"("Val(Sgnl)"=w745) -> ()  [unwired: 2 in, 2 out]
          }
          frame True {
          }
        }
      }
      event "Round T1 X": Value Change {
        n415 = event-data() -> ()  [unwired: 7 out]
        n416 = local read "BD 1 Frequency 1 (MHz)"() -> (w761:dbl)
        n417 = Round To Nearest(number=w761) -> (nearest integer value=w760:dbl)
        n418 = property on="BD 1 Frequency 1 (MHz)" class="DigNum (strict)"("Val(Sgnl)"=w760) -> ()  [unwired: 2 in, 2 out]
      }
      event "Restart RF": Value Change {
        n419 = event-data() -> ()  [unwired: 7 out]
        n420 = xnode "Read/Write Control"("FPGA VI Reference In"=w799, "error in"=w794, "FPGA Controls  RF Box"=FALSE) -> ("FPGA VI Reference Out"=w798:T19, "error out"=w793:errorcluster)
        n421 = local read "Y RF Amplitude Limits (%)"() -> (w774:T16)
        n422 = local read "X RF Amplitude Limits (%)"() -> (w775:T16)
        n423 = local read "X RF Frequency Limits (MHz)"() -> (w777:T16)
        n424 = local read "Y RF Frequency Limits (MHz)"() -> (w776:T16)
        n425 = xnode "Read/Write Control"("FPGA VI Reference In"=w798, "error in"=w793, "Direct RF Box  Communication"=TRUE) -> ("FPGA VI Reference Out"=w797:T19, "error out"=w792:errorcluster)
        n426 = local read "BD 2 Frequency 3 (MHz)"() -> (w784:dbl)
        n427 = local read "BD 2 Frequency 2 (MHz)"() -> (w785:dbl)
        n428 = local read "BD 1 Frequency 3 (MHz)"() -> (w788:dbl)
        n429 = local read "BD 1 Frequency 1 (MHz)"() -> (w789:dbl)
        n430 = local read "BD 2 Frequency 1 (MHz)"() -> (w786:dbl)
        n431 = local read "BD 1 Frequency 2 (MHz)"() -> (w787:dbl)
        n432 = call "Initialize RF boards - interlace 3.vi"("error in"=w792, "FPGA VI Reference In"=w797) -> ("error out"=w791:errorcluster, "FPGA VI Reference Out"=w796:T19)
        n433 = local read "BD 2 Amplitude 2 (%)"() -> (w779:dbl)
        n434 = local read "BD 2 Amplitude 1 (%)"() -> (w780:dbl)
        n435 = local read "BD 2 Amplitude 3 (%)"() -> (w778:dbl)
        n436 = local read "BD 1 Amplitude 3 (%)"() -> (w783:dbl)
        n437 = local read "BD 1 Amplitude 1 (%)"() -> (w782:dbl)
        n438 = local read "BD 1 Amplitude 2 (%)"() -> (w781:dbl)
        n439 = call "set RF board frequency - interlace.vi"("Board 2 Frequency Limits"=w776, "Board 1 Frequency Limits"=w777, "error in"=w791, "FPGA VI Reference In"=w796, "Board 2 Frequency 3 (MHz)"=w784, "Board 1 Frequency 3 (MHz)"=w788, "Board 2 Frequency 2 (MHz)"=w785, "Board 2 Frequency 1 (MHz)"=w786, "Board 1 Frequency 2 (MHz)"=w787, "Board 1 Frequency 1  (MHz)"=w789) -> ("error out"=w790:errorcluster, "FPGA VI Reference Out"=w795:T19)
        n440 = call "set RF board amplitude - interlace.vi"("Board 2 Amplitude Limits"=w774, "Board 1 Amplitude Limits"=w775, "error in"=w790, "FPGA VI Reference In"=w795, "Board 2 Amplitude 3 (%)"=w778, "Board 1 Amplitude 3 (%)"=w783, "Board 2 Amplitude 2 (%)"=w779, "Board 2 Amplitude 1 (%)"=w780, "Board 1 Amplitude 2 (%)"=w781, "Board 1 Amplitude 1 (%)"=w782) -> ("error out"=w767:errorcluster, "FPGA VI Reference Out"=w771:T19)
        n441 = xnode "Read/Write Control"("FPGA VI Reference In"=w771, "error in"=w767, "Direct RF Box  Communication"=FALSE) -> ("FPGA VI Reference Out"=w770:T19, "error out"=w769:errorcluster)
        n442 = flat-sequence {
          tunnel: w769 -> [w800]
          tunnel: [w800] -> w768
          frame #0 {
            n443 = Wait (ms)(milliseconds to wait=u32 50) -> ()  [unwired: 1 out]
          }
        }
        n444 = xnode "Read/Write Control"("FPGA VI Reference In"=w770, "error in"=w768, "FPGA Controls  RF Box"=TRUE) -> ("error out"=w763:errorcluster)  [unwired: 1 out]
        n445 = property on="Restart RF" class="Bool (strict)"(error in=w763, "Value"=FALSE ("Restart RF")) -> (error out=w762:errorcluster)  [unwired: 1 in, 1 out]
      }
      event "Round T2 X": Value Change {
        n446 = event-data() -> ()  [unwired: 7 out]
        n447 = local read "BD 1 Frequency 2 (MHz)"() -> (w803:dbl)
        n448 = Round To Nearest(number=w803) -> (nearest integer value=w802:dbl)
        n449 = property on="BD 1 Frequency 2 (MHz)" class="DigNum (strict)"("Val(Sgnl)"=w802) -> ()  [unwired: 2 in, 2 out]
      }
      event "Stop All": Value Change {
        n450 = event-data() -> ()  [unwired: 7 out]
        n451 = call "hamilton_controller.vi"("action"=T21."DISCONNECT") -> ()  [unwired: 10 in, 1 out]
        n452 = local read "Stop All"() -> (w806:bool)
      }
      event "Delayed Interlace Start": Value Change {
        n453 = event-data() -> ()  [unwired: 7 out]
        n454 = flat-sequence {
          frame #0 {
            n455 = Multiply(x="Delay to Interlace (s)", y=1000.0) -> (x*y=w809:dbl)
            n456 = Wait (ms)(milliseconds to wait=w809) -> ()  [unwired: 1 out]
          }
          frame #1 {
            n457 = property on="Green laser mode" class="RadioBtnsControl (strict)"("Val(Sgnl)"=enum32{"Laser ON", "Laser OFF", "Interlace"}."Interlace" ("Value (Signaling)")) -> ()  [unwired: 2 in, 2 out]
          }
        }
      }
      event "BD 1 Amplitude 1 (%)", "BD 1 Amplitude 2 (%)", "BD 1 Amplitude 3 (%)", "BD 2 Amplitude 1 (%)", "BD 2 Amplitude 2 (%)", "BD 2 Amplitude 3 (%)", "Trap 1 ON", "Trap 2 ON", "Trap 3 ON", "Feedback On/Off", "All FB On/Off": Value Change {
        w833 = i16 1 ("f")
        n458 = event-data() -> ()  [unwired: 7 out]
        n459 = local write "Trap 1 (ON/OFF)"("Trap 1 ON") -> ()
        n460 = local write "Trap 2 (ON/OFF)"("Trap 2 ON") -> ()
        n461 = Boolean To (0,1)(Boolean="Trap 3 ON") -> (0, 1=w834:i16)
        n462 = Boolean To (0,1)(Boolean="Trap 1 ON") -> (0, 1=w835:i16)
        n463 = Boolean To (0,1)(Boolean="Trap 2 ON") -> (0, 1=w836:i16)
        n464 = Select(t=w836, s="Trap ON/OFF X or Y Amp?", f=w833) -> (s? t:f=w831:i16)
        n465 = Select(t=w835, s="Trap ON/OFF X or Y Amp?", f=w833) -> (s? t:f=w832:i16)
        n466 = Select(t=w834, s="Trap ON/OFF X or Y Amp?", f=w833) -> (s? t:f=w830:i16)
        n467 = Select(t=w833, s="Trap ON/OFF X or Y Amp?", f=w836) -> (s? t:f=w828:i16)
        n468 = Select(t=w833, s="Trap ON/OFF X or Y Amp?", f=w835) -> (s? t:f=w829:i16)
        n469 = Select(t=w833, s="Trap ON/OFF X or Y Amp?", f=w834) -> (s? t:f=w827:i16)
        n470 = And(x="All FB On/Off", y="Feedback On/Off") -> (x .and. y?=w825:cluster{"Set 1":bool, "Set 2":bool})
        n471 = local read "BD 1 Amplitude 1 (%)"() -> (w845:dbl)
        n472 = local read "BD 1 Amplitude 2 (%)"() -> (w844:dbl)
        n473 = local read "BD 1 Amplitude 3 (%)"() -> (w843:dbl)
        n474 = Unbundle By Name(w825) -> ("Set 1"=w820:bool, "Set 2"=w817:bool)
        n475 = local read "Y RF Amplitude Limits (%)"() -> (w813:T16)
        n476 = local read "X RF Amplitude Limits (%)"() -> (w814:T16)
        n477 = local read "BD 2 Amplitude 1 (%)"() -> (w846:dbl)
        n478 = local read "BD 2 Amplitude 2 (%)"() -> (w847:dbl)
        n479 = local read "BD 2 Amplitude 3 (%)"() -> (w848:dbl)
        n480 = And(x="Trap 2 ON", y=w817) -> (x .and. y?=w815:bool)
        n481 = And(x="Trap 1 ON", y=w820) -> (x .and. y?=w818:bool)
        n482 = Multiply(x=w832, y=w845) -> (x*y=w840:dbl)
        n483 = Multiply(x=w844, y=w831) -> (x*y=w838:dbl)
        n484 = Multiply(x=w843, y=w830) -> (x*y=w839:dbl)
        n485 = Multiply(x=w846, y=w829) -> (x*y=w849:dbl)
        n486 = Multiply(x=w847, y=w828) -> (x*y=w850:dbl)
        n487 = Multiply(x=w848, y=w827) -> (x*y=w851:dbl)
        n488 = call "set RF board amplitude - interlace.vi"("Board 2 Amplitude Limits"=w813, "Board 1 Amplitude Limits"=w814, "error in"=w841, "FPGA VI Reference In"=w842, "Board 2 Amplitude 3 (%)"=w851, "Board 1 Amplitude 3 (%)"=w839, "Board 2 Amplitude 2 (%)"=w850, "Board 2 Amplitude 1 (%)"=w849, "Board 1 Amplitude 2 (%)"=w838, "Board 1 Amplitude 1 (%)"=w840) -> ("error out"=w822:errorcluster, "FPGA VI Reference Out"=w823:T19)
        n489 = xnode "Read/Write Control"("FPGA VI Reference In"=w823, "error in"=w822, "FB On/Off Set 1"=w818, "FB On/Off Set 2"=w815) -> ("error out"=w821:errorcluster)  [unwired: 1 out]
      }
      event "Load parameters": Value Change {
        n490 = event-data() -> ()  [unwired: 7 out]
        n491 = property on="Saved AOD Raster Scan Parameter Sets" class="Arr (strict)"() -> ("Index Values"=w862:u32[])  [unwired: 2 in, 2 out]
        n492 = Index Array(array=w862, index=0) -> (element=w859:u32)
